vi "setPerturbance.vi"(0 "Interface in":T1, 5 "pertAmp":sgl, 7 "pertFreq":sgl, 9 "controlFreq":sgl, 11 "error in (no error)":errorcluster) -> (4 "Interface out":T1, 15 "error out":errorcluster)   [LabVIEW 2017, in "BuckBoostInterface.lvlib"]
uses:
  BuckBoostInterface.lvlib
  Interface.ctl
  <instrlib>/_niInstr/Instruction Framework/v1/Host/Instruction Target/niInstr Instruction Target v1 Host.lvclass
  <instrlib>/_niInstr/Instruction Framework/v1/Host/Instruction Framework Context/niInstr Instruction Framework Context v1 Host.lvclass
  <vilib>/NI/JSON Support for LabVIEW/JSON Data Classes/JSON Numeric/JSON Numeric.lvclass
  C:/Program Files (x86)/National Instruments/LabVIEW 2017/vi.lib/NI/JSON Support for LabVIEW/JSON Data Classes/JSON Datatype/JSON Null.lvclass
  <vilib>/NI/JSON Support for LabVIEW/JSON Data Classes/JSON Numeric/New JSON Numeric.vi
  <vilib>/NI/JSON Support for LabVIEW/JSON Data Classes/JSON Object/New JSON Object (Empty).vi
  <vilib>/NI/JSON Support for LabVIEW/JSON Data Classes/JSON Object/Insert Key Value Pair (Multi).vi
  <vilib>/NI/JSON Support for LabVIEW/JSON Data Classes/JSON Helper/Parsing/Parse Value.vi
  <vilib>/NI/JSON Support for LabVIEW/JSON Data Classes/JSON Helper/To More Specific Type (Object).vi
  <vilib>/NI/JSON Support for LabVIEW/JSON Data Classes/JSON Datatype/JSON Null.lvclass
  <vilib>/NI/JSON Support for LabVIEW/JSON Data Classes/JSON Object/JSON Object.lvclass
  <vilib>/NI/JSON Support for LabVIEW/JSON Data Classes/JSON Helper/JSON Helper.lvclass
  C:/Program Files (x86)/National Instruments/LabVIEW 2017/vi.lib/NI/JSON Support for LabVIEW/JSON Data Classes/JSON Basic Type/JSON Literal.lvclass
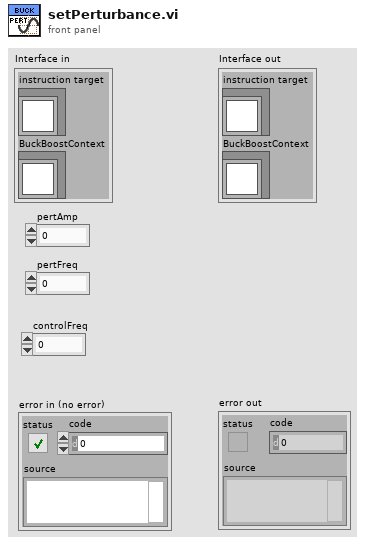
[diagram p1: front panel]
types:
  T1 = typedef "BuckBoostInterface.lvlib/Interface.ctl" = cluster{"instruction target":refnum<class "niInstr Instruction Target v1 Host.lvclass">, "BuckBoostContext":refnum<class "niInstr Instruction Framework Context v1 Host.lvclass">}
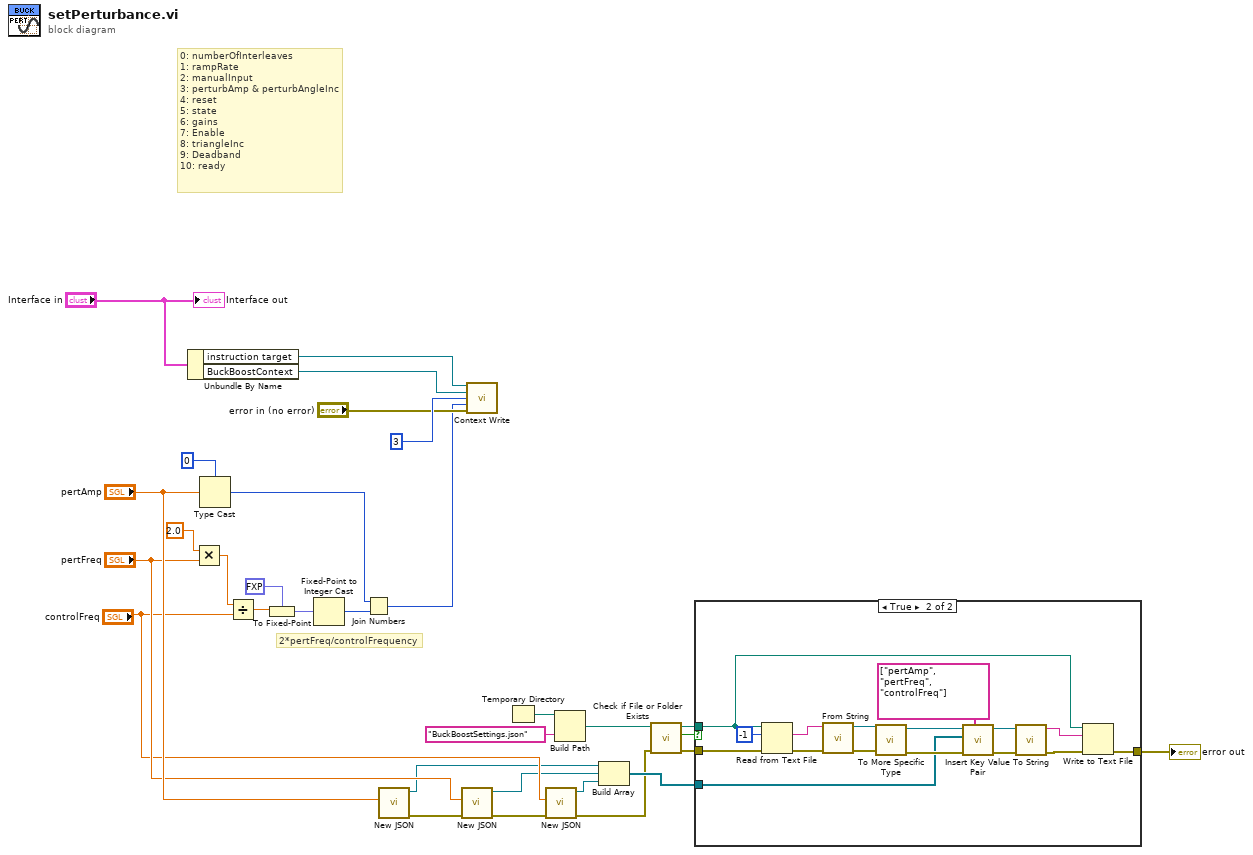
[diagram p0: block diagram]
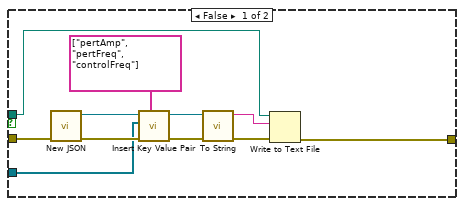
[diagram p2: hidden frame]
diagram:
  # "2*pertFreq/controlFrequency"
  # "0: numberOfInterleaves\n1: rampRate\n2: manualInput\n3: perturbAmp & perturbAngleInc\n4: reset\n5: state\n6: gains\n7: Enable\n8: triangleInc\n9: Deadband\n10: ready"
  n1 = Unbundle By Name("Interface in") -> ("instruction target"=w27:refnum<class "niInstr Instruction Target v1 Host.lvclass">, "BuckBoostContext"=w26:refnum<class "niInstr Instruction Framework Context v1 Host.lvclass">)
  n2 = Multiply(x=2.0, y="pertFreq") -> (x*y=w24:dbl)
  n3 = Type Cast(type=u32 0, x="pertAmp") -> (*(type *) &x=w19:u32)
  n4 = Divide(x=w24, y="controlFreq") -> (x/y=w23:dbl)
  n5 = To Fixed-Point(fixed-point type=fxp<+/-,16,0> 0.0 ("Data"), number=w23) -> (fixed-point=w21:fxp<+/-,16,0>)
  n6 = Fixed-Point to Integer Cast(1:w21) -> (0:w20:i16)
  n7 = Join Numbers(hi=w19, lo=w20) -> ((hi.lo)=w18:u64)
  n8 = call-poly <vilib>:"New JSON.vi"("value"="pertAmp") -> ("error out"=w9:errorcluster, "JSON String out"=w5:refnum<class "JSON Numeric.lvclass">)  [unwired: 9 in]
  n9 = call-poly <vilib>:"New JSON.vi"("error in (no error)"=w9, "value"="pertFreq") -> ("error out"=w10:errorcluster, "JSON String out"=w4:refnum<class "JSON Numeric.lvclass">)  [unwired: 8 in]
  n10 = call <instrlib>:"Context Write.vi"("instruction target in"=w27, "context in"=w26, "address"=u64 3, "data"=w18, "error in"="error in (no error)") -> ()  [unwired: 8 in, 3 out]
  n11 = Temporary Directory() -> (w17:path)
  n12 = call-poly <vilib>:"New JSON.vi"("error in (no error)"=w10, "value"="controlFreq") -> ("error out"=w1:errorcluster, "JSON String out"=w3:refnum<class "JSON Numeric.lvclass">)  [unwired: 8 in]
  n13 = Build Path(base path=w17, name or relative path="BuckBoostSettings.json") -> (appended path=w15:path)
  n14 = Build Array(w5, w4, w3) -> (w2:refnum<class "JSON Numeric.lvclass">[])
  n15 = call <vilib>:"Check if File or Folder Exists.vi"("error in (no error)"=w1, "path"=w15) -> ("error out"=w12:errorcluster, "file or folder exists?"=w13:bool, "dup path"=w14:path)  [unwired: 7 in]
  n16 = case shown="True" w13 {
    tunnel: w14 -> [w39 w51]
    tunnel: w12 -> [w42 w52]
    tunnel: [w38 w46] -> w11
    tunnel: w2 -> [w33 w45]
    frame False {
      n17 = call-poly <vilib>:"New JSON.vi"("error in (no error)"=w42) -> ("error out"=w40:errorcluster, "JSON Object out"=w41:refnum<class "JSON Object.lvclass">)  [unwired: 9 in]
      n18 = call-poly <vilib>:"Insert Key Value Pair.vi"("keys"=string[] ["pertAmp", "pertFreq", "controlFreq"], "error in (no error)"=w40, "values"=w33, "JSON Object in"=w41) -> ("error out"=w37:errorcluster, "JSON Object out"=w34:refnum<class "JSON Object.lvclass">)  [unwired: 5 in, 1 out]
      n19 = call-dynamic "To String.vi"("error in (no error)"=w37, "JSON Object in"=w34) -> ("error out"=w36:errorcluster, "String"=w35:string)  [unwired: 8 in]
      n20 = Write to Text File(file (use dialog)=w39, text=w35, error in=w36) -> (error out=w38:errorcluster)  [unwired: 1 in, 2 out]
    }
    frame True {
      n21 = Read from Text File(file (use dialog)=w51, count=-1, error in=w52) -> (text=w58:string, error out=w53:errorcluster)  [unwired: 1 in, 2 out]
      n22 = call <vilib>:"From String.vi"("error in (no error)"=w53, "JSON String"=w58) -> ("error out"=w57:errorcluster, "JSON out"=w56:refnum<class "JSON Null.lvclass">)  [unwired: 8 in]
      n23 = call-poly <vilib>:"To More Specific Type.vi"("error in (no error)"=w57, "JSON Datatype in"=w56) -> ("error out"=w54:errorcluster, "JSON Datatype out"=w55:refnum<class "JSON Object.lvclass">)  [unwired: 8 in]
      n24 = call-poly <vilib>:"Insert Key Value Pair.vi"("keys"=string[] ["pertAmp", "pertFreq", "controlFreq"], "error in (no error)"=w54, "values"=w45, "JSON Object in"=w55) -> ("error out"=w48:errorcluster, "JSON Object out"=w50:refnum<class "JSON Object.lvclass">)  [unwired: 5 in, 1 out]
      n25 = call-dynamic "To String.vi"("error in (no error)"=w48, "JSON Object in"=w50) -> ("error out"=w47:errorcluster, "String"=w49:string)  [unwired: 8 in]
      n26 = Write to Text File(file (use dialog)=w51, text=w49, error in=w47) -> (error out=w46:errorcluster)  [unwired: 1 in, 2 out]
    }
  }
  "error out" <- w11
  "Interface out" <- "Interface in"
